vi "Init Device.vi"(10 "Home type value :\n0 use MZ switch and encoder Index\n1 use current position as HOME\n2 use MZ switch only\n3 use EoR- switch and encoder Index\n4 use EoR- switch only":i32, 11 "SerialPort":u8) -> (0 "error out":errorcluster, 3 "VISA Refnum out":refnum<visa-resource-name>)   [LabVIEW 2020, in "SMC100.lvlib"]
uses:
  SMC100.lvlib
  SMC100-Controller-Drivers/SMC100.llb/enter / leave disable state.vi
  SMC100-Controller-Drivers/SMC100.llb/enter / leave configuration state.vi
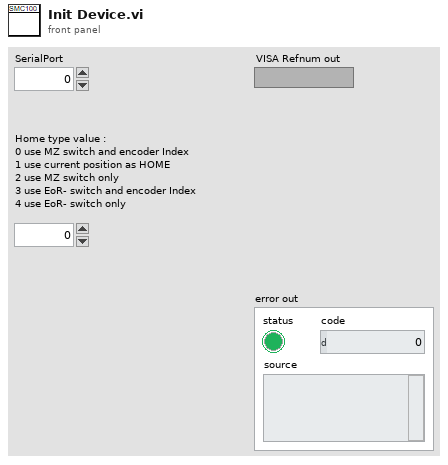
[diagram p1: front panel]
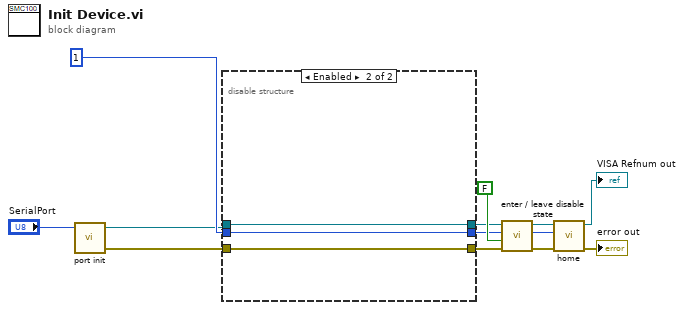
[diagram p0: block diagram]
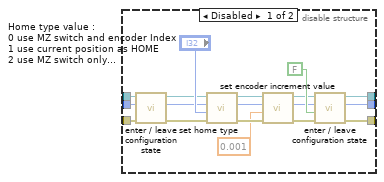
[diagram p2: hidden frame]
diagram:
  n1 = call "port init.vi"("SerialPort"="SerialPort") -> ("error out"=w3:errorcluster, "Visa Handle"=w1:refnum<visa-resource-name>)  [unwired: 3 in]
  n2 = disable-structure shown="Enabled" {
    disable-tunnel: [w27 w32] -> w6
    disable-tunnel: w3 -> [w24 w32]
    disable-tunnel: w1 -> [w23 w34]
    disable-tunnel: 1 ("Axis in") -> [w22 w33]
    disable-tunnel: [w16 w34] -> w5
    disable-tunnel: [w15 w33] -> w4
    frame Disabled {
      n3 = call "enter / leave configuration state.vi"("error in"=w24, "Axis in"=w22, "VISA handle in"=w23) -> ("error out"=w25:errorcluster, "Axis out"=w20:i32, "VISA handle out"=w21:refnum<visa-resource-name>)  [unwired: 5 in, 1 out]
      n4 = call "set home type.vi"("error in"=w25, "Home type value :\n0 use MZ switch and encoder Index\n1 use current position as HOME\n2 use MZ switch only\n3 use EoR- switch and encoder Index\n4 use EoR- switch only"="Home type value :\n0 use MZ switch and encoder Index\n1 use current position as HOME\n2 use MZ switch only\n3 use EoR- switch and encoder Index\n4 use EoR- switch only", "Axis in"=w20, "VISA Handle in"=w21) -> ("error out"=w30:errorcluster, "Axis out"=w28:i32, "VISA Handle out"=w18:refnum<visa-resource-name>)  [unwired: 2 in, 1 out]
      n5 = call "set encoder increment value.vi"("error in"=w30, "Encoder increment value (units)"=0.001, "Axis in"=w28, "VISA Handle in"=w18) -> ("error out"=w29:errorcluster, "Axis out"=w14:i32, "VISA Handle out"=w17:refnum<visa-resource-name>)  [unwired: 2 in, 1 out]
      n6 = call "enter / leave configuration state.vi"("error in"=w29, "enter configuration state (True)"=FALSE, "Axis in"=w14, "VISA handle in"=w17) -> ("error out"=w27:errorcluster, "Axis out"=w15:i32, "VISA handle out"=w16:refnum<visa-resource-name>)  [unwired: 4 in, 1 out]
    }
    frame Enabled {
    }
  }
  n7 = call "enter / leave disable state.vi"("error in"=w6, "enter disable state (True)"=FALSE, "Axis in"=w4, "VISA handle in"=w5) -> ("error out"=w12:errorcluster, "Axis out"=w7:i32, "VISA handle out"=w8:refnum<visa-resource-name>)  [unwired: 4 in, 1 out]
  n8 = call "home.vi"("error in"=w12, "Axis in"=w7, "VISA Handle in"=w8) -> ("error out"=→"error out":errorcluster, "VISA Handle out"=→"VISA Refnum out":refnum<visa-resource-name>)  [unwired: 3 in, 2 out]
